vi "FXP NILIA_CIC_Stage.vi"(8 "decimate factor":i16, 9 "New Data":bool, 11 "input":i64) -> (1 "Data Ready":bool, 3 "output":i64)   [LabVIEW 2009]
panel:
  in  "count":i16
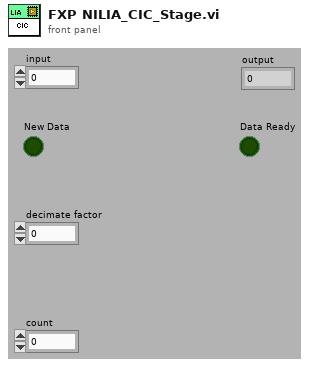
[diagram p1: front panel]
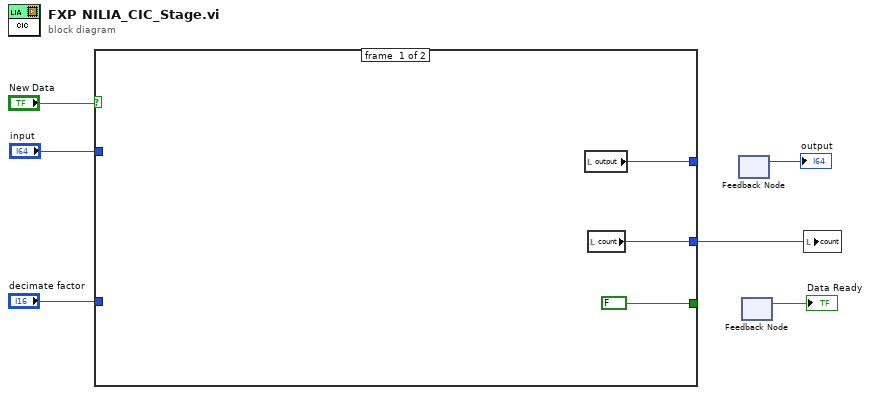
[diagram p0: block diagram]
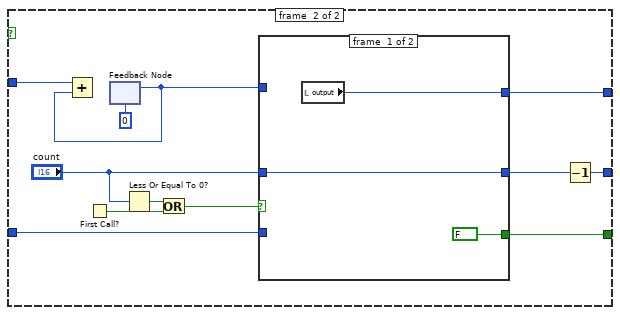
[diagram p2: hidden frame]
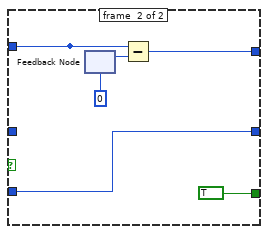
[diagram p3: hidden frame]
diagram:
  n1 = case shown="True" "New Data" {
    tunnel: [w10 w24] -> w4
    tunnel: "decimate factor" -> [_ w23]
    tunnel: [w11 w21] -> w7
    tunnel: "input" -> [_ w15]
    tunnel: [FALSE ("Data Ready") w14] -> w2
    frame #0 {
      n2 = local read "output"() -> (w10:i64)
      n3 = local read "count"() -> (w11:i16)
    }
    frame #1 {
      n4 = First Call?() -> (First Call?: T/F=w19:bool)
      n5 = feedback #1(i64 0) -> (w12:i64)
      n6 = Add(x=w15, y=w12) -> (x+y=w13:i64)
      n7 = Less Or Equal To 0?(x="count") -> (x <= 0?=w20:bool)
      n8 = Or(x=w20, y=w19) -> (x .or. y?=w18:bool)
      n9 = case shown="True" w18 {
        tunnel: w12 -> [_ w29]
        tunnel: [w26 w28] -> w24
        tunnel: "count" -> [w27 _]
        tunnel: [w27 w33] -> w22
        tunnel: w23 -> [_ w33]
        tunnel: [FALSE ("Data Ready") TRUE ("Data Ready")] -> w14
        frame #0 {
          n10 = local read "output"() -> (w26:i64)
        }
        frame #1 {
          n11 = feedback #2(i64 0) -> (w32:i64)
          n12 = Subtract(x=w29, y=w32) -> (x-y=w28:i64)
        }
      }
      n13 = Decrement(x=w22) -> (x-1=w21:i16)
    }
  }
  n14 = feedback #3() -> (→"output":i64)  [unwired: 1 in]
  n15 = feedback #4() -> (→"Data Ready":bool)  [unwired: 1 in]
  n16 = local write "count"(w7) -> ()
